vi "DVR Destroy.vi"(8 "error in (no error)":errorcluster) -> (0 "error out":errorcluster)   [LabVIEW 2015]
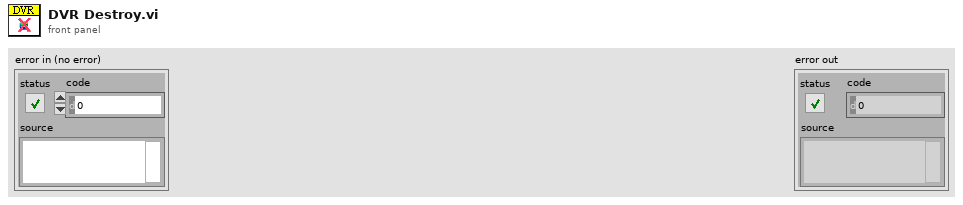
[diagram p1: front panel]
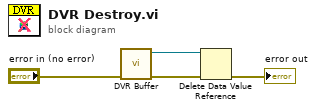
[diagram p0: block diagram]
diagram:
  n1 = call "DVR Buffer.vi"("error in (no error)"="error in (no error)") -> ("error out"=w1:errorcluster, "DVR Out"=w3:refnum<data-value>)  [unwired: 9 in]
  n2 = Delete Data Value Reference(data value reference=w3, error in=w1) -> (error out=→"error out":errorcluster)  [unwired: 1 out]
